vi "SelectExample.vi"() -> ()   [LabVIEW 2017]
uses:
  <vilib>/addons/database/Auxilliary.llb/DB Tools Cursor Type.ctl
  <vilib>/addons/database/Connection.llb/DB Tools Open Connec (Path).vi
  <vilib>/addons/database/Connection.llb/Conn Execute.vi
  <vilib>/addons/database/Recordset.llb/Rec Fetch Recordset Data (R).vi
  <vilib>/addons/database/Recordset.llb/Rec Destroy - Connection.vi
  <vilib>/addons/database/NI_Database_API.lvlib
panel:
  out "recordset data":variant[][](array[variant])
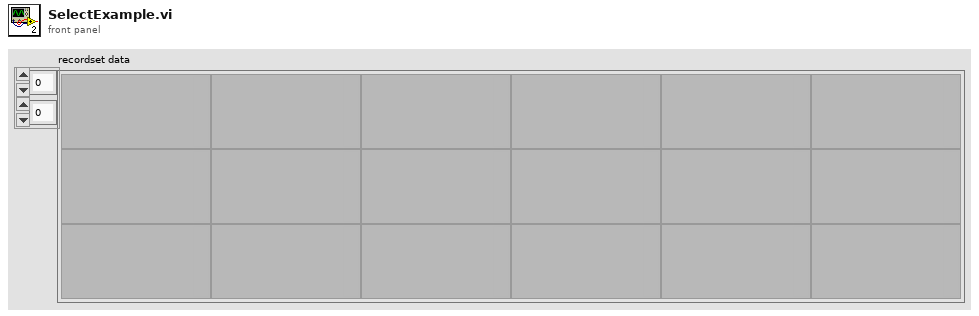
[diagram p1: front panel]
types:
  T1 = typedef "NI_Database_API.lvlib/DB Tools Cursor Type.ctl" = enum16{"forward-only", "keyset", "dynamic", "static"}
  T2 = typedef "NI_Database_API.lvlib/Conn ObjectReference.ctl" = refnum<k1>
  T3 = typedef "NI_Database_API.lvlib/Rec ObjectReference.ctl" = refnum<k1>
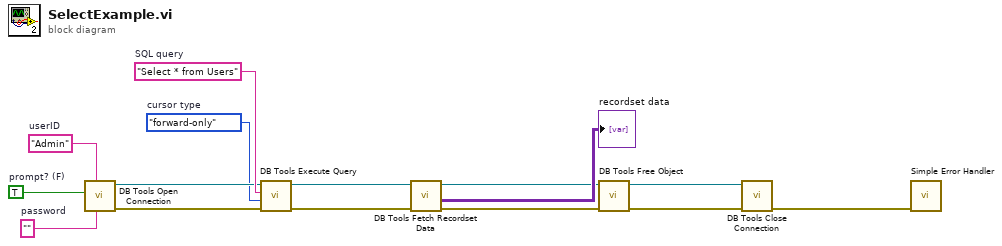
[diagram p0: block diagram]
diagram:
  w5 = DB_Tools_Cursor_Type."forward-only"  # cursor type
  w10 = "Select * from Users"  # SQL query
  w13 = ""  # password
  w14 = TRUE  # prompt? (F)
  w15 = "Admin"  # userID
  n1 = call-poly <vilib>:"DB Tools Open Connection.vi"("password"=w13, "userID"=w15, "prompt? (F)"=w14) -> ("error out"=w9:errorcluster, "connection reference"=w7:T2)  [unwired: 5 in]
  n2 = call-poly <vilib>:"DB Tools Execute Query.vi"("error in (no error)"=w9, "cursor type"=w5, "SQL query"=w10, "connection reference"=w7) -> ("error out"=w8:errorcluster, "recordset reference"=w11:T3)  [unwired: 4 in]
  n3 = call-poly <vilib>:"DB Tools Fetch Recordset Data.vi"("error in (no error)"=w8, "recordset reference"=w11) -> ("error out"=w2:errorcluster, "recordset data"=→"recordset data":variant[][], "recordset reference out"=w4:T3)  [unwired: 3 in]
  n4 = call-poly <vilib>:"DB Tools Free Object.vi"("error in (no error)"=w2, "recordset reference"=w4) -> ("error out"=w1:errorcluster, "connection reference"=w3:T2)  [unwired: 8 in]
  n5 = call <vilib>:"DB Tools Close Connection.vi"("error in (no error)"=w1, "connection reference"=w3) -> ("error out"=w6:errorcluster)  [unwired: 5 in]
  n6 = call <vilib>:"Simple Error Handler.vi"("error in (no error)"=w6) -> ()  [unwired: 4 in, 5 out]
